vi "Load_SampleImages.vi"(8 "error in":errorcluster caption="entrée d'erreur") -> (0 "error out":errorcluster caption="sortie d'erreur", 3 "Image (RGB)":cluster{"Tableau":string[][]}[](array[cluster]))   [LabVIEW 2020]
doc: "Scikit-learn also embed a couple of sample JPEG images published under Creative Commons license by their authors. Those images can be useful to test algorithms and pipeline on 2D data.\n\nImages name : china.jpg, flower.jpg\n\nThe image as a numpy array : height x width x color(RGB)"
uses:
  Load_SampleImages.lvclass
panel:
  out "Load_SampleImages.lvclass":refnum<class "Load_SampleImages.lvclass">
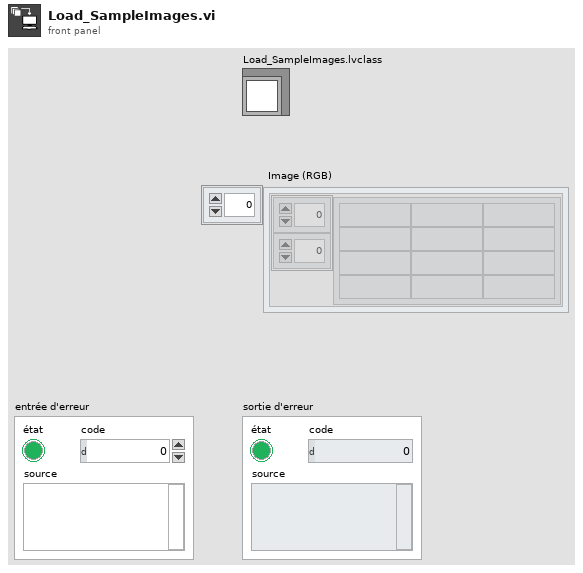
[diagram p1: front panel]
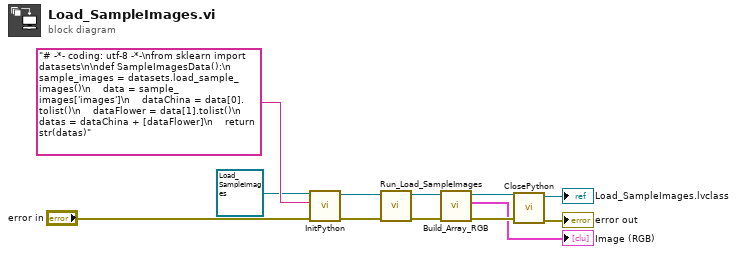
[diagram p0: block diagram]
diagram:
  n1 = call-dynamic "InitPython.vi"("error in (no error)"="error in", "Python Instruction"="# -*- coding: utf-8 -*-\nfrom sklearn import datasets\n\ndef SampleImagesData():\n    sample_images = datasets.load_sample_images()\n    data = sample_images['images']\n    dataChina = data[0].tolist()\n    dataFlower = data[1].tolist()\n    datas = dataChina + [dataFlower]\n    return str(datas)", "Scikit-learn en entrée"=refnum<class "Load_SampleImages.lvclass"> refnum ("Load_SampleImages.lvclass")) -> ("error out"=w7:errorcluster, "Scikit-learn en sortie"=w6:refnum<class "Load_SampleImages.lvclass">)  [unwired: 7 in]
  n2 = call-dynamic "Run_Load_SampleImages.vi"("error in (no error)"=w7, "Load_SampleImages.lvclass"=w6) -> ("error out"=w4:errorcluster, "Load_SampleImages.lvclass"=w5:refnum<class "Load_SampleImages.lvclass">)  [unwired: 8 in]
  n3 = call-dynamic "Build_Array_RGB.vi"("error in (no error)"=w4, "Load_SampleImages.lvclass"=w5) -> ("error out"=w2:errorcluster, "Image (RGB)"=→"Image (RGB)":cluster{"Tableau":string[][]}[], "Load_SampleImages.lvclass"=w3:refnum<class "Load_SampleImages.lvclass">)  [unwired: 7 in]
  n4 = call-dynamic "ClosePython.vi"("error in (no error)"=w2, "Scikit-learn en entrée"=w3) -> ("error out"=→"error out":errorcluster, "Scikit-learn en sortie"=→"Load_SampleImages.lvclass":refnum<class "Load_SampleImages.lvclass">)  [unwired: 8 in]
